vi "Proyecto2.vi"() -> ()   [LabVIEW 2015]
uses:
  <vilib>/Utility/NIReport.llb/image depth.ctl
  <vilib>/MakerHub/LINX/Public/Peripherals/PWM/PWM Set Duty Cycle 1 Chan.vi
  <vilib>/MakerHub/LINX/Public/Peripherals/Digital/Digital Write 1 Chan.vi
  <vilib>/MakerHub/LINX/Public/Peripherals/Digital/Digital Write N Chans.vi
  <vilib>/MakerHub/LINX/Private/Local IO/LinxDigitalWrite.vi
  <vilib>/MakerHub/LINX/Public/Utilities/Check Channel.vi
  <vilib>/MakerHub/LINX/Public/Utilities/Open Serial.vi
  <vilib>/MakerHub/LINX/Public/Peripherals/PWM/PWM Set Duty Cycle N Chans.vi
  <vilib>/MakerHub/LINX/Private/Utilties/Generate Error.vi
  <vilib>/Utility/NIReport.llb/Append Report Text (str wrap).vi
  <vilib>/printing/OpenHTMLReport.llb/Open HTML Report in Browser (Refnum).vi
  <vilib>/Utility/NIReport.llb/NI_report.lvclass
  <vilib>/MakerHub/LINX/LMH-LINX.lvlib
  <vilib>/Utility/NIReport.llb/NI_ReportGenerationCore.lvlib
panel:
  out "Temporary HTML file created":path
  in  "Header":string="Example Report with Images"
  in  "Body":string="<tab>This is an example of some of the things that you can do with HTML reports. <newline> <tab>Above is an image of a Waveform Chart Control.  Below is a horizontal line.  Below that is a link to NI's homepage.<newline>"
  out "Grafica de  distancia entre vehiculo objeto\ndurante el viaje":dbl(graph)
  in  "stop":bool
  out "Velocidad del motor (Escala 0 a 1)":dbl(slide) scale=0.0..1.0
  out "Vehiculo avanzando hacia adelante":bool
  out "Se mantiene a una distancia segura":bool
  out "Precaucion! Bajando a velocidad segura":bool
  out "Distancia entre conductor y vehiculo delantero":dbl
  in  "Echo Pin (DI)":u8
  in  "Trigger":u8
  in  "Serial Port":refnum<visa-resource-name>="N/A"
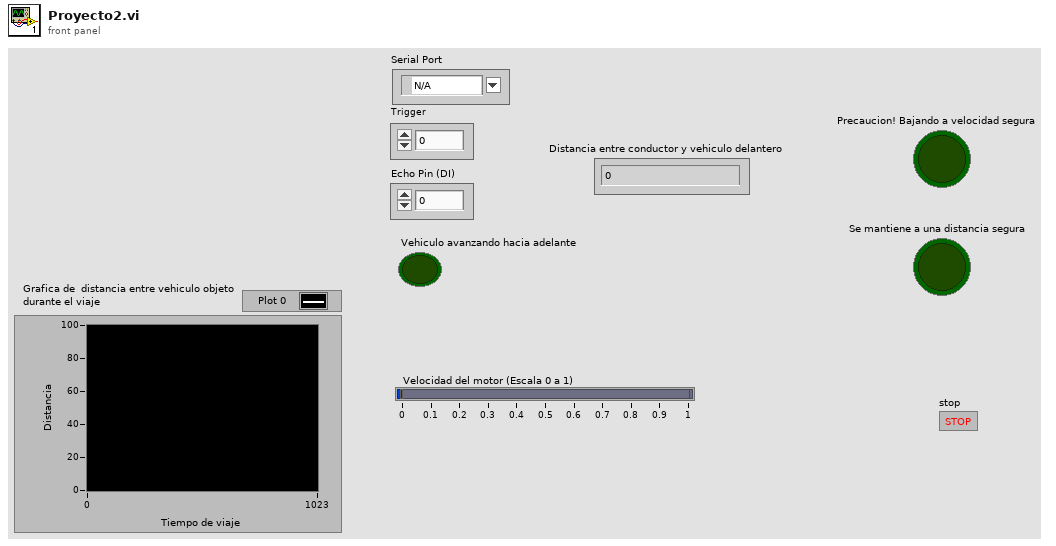
[diagram p1: front panel]
types:
  T1 = typedef "LMH-LINX.lvlib/LINX Ref.ctl" = cluster{"IO":T2, "Interface":T3, "LINX Device Config":T4}
  T2 = typedef "LMH-LINX.lvlib/Platform.ctl" = enum16{"Remote", "Local"}
  T3 = typedef "LMH-LINX.lvlib/Interface.ctl" = enum16{"Serial", "TCP"}
  T4 = typedef "LMH-LINX.lvlib/Device.lvlib/LINX Device Config.ctl" = cluster{"Interface":T3, "COM Port":refnum<visa-resource-name>, "TCP Configuration":T5, "Device Family":u8, "Device ID":u8, "Device Name":string, "TCP Ref":refnum<k5>, "Channels":T6}
  T5 = typedef "LMH-LINX.lvlib/Device.lvlib/TCP Config.ctl" = cluster{"IP Address":string, "Port":u16}
  T6 = typedef "LMH-LINX.lvlib/Channels.ctl" = cluster{"DI":u8[], "DO":u8[], "AI":u8[], "AO":u8[], "PWM":u8[], "QE":u8[], "UART":u8[], "I2C 2":u8[], "SPI":u8[], "CAN":u8[], "Servo":u8[], "AI Ref (V)":dbl, "AI Resolution (Bits)":u8, "AO Ref (V)":dbl, "AO Resolution (Bits)":u8}
  T7 = enum16{"Standard Report", "HTML", "Word", "Excel"}
  T8 = typedef "NI_ReportGenerationCore.lvlib/image depth.ctl" = u16
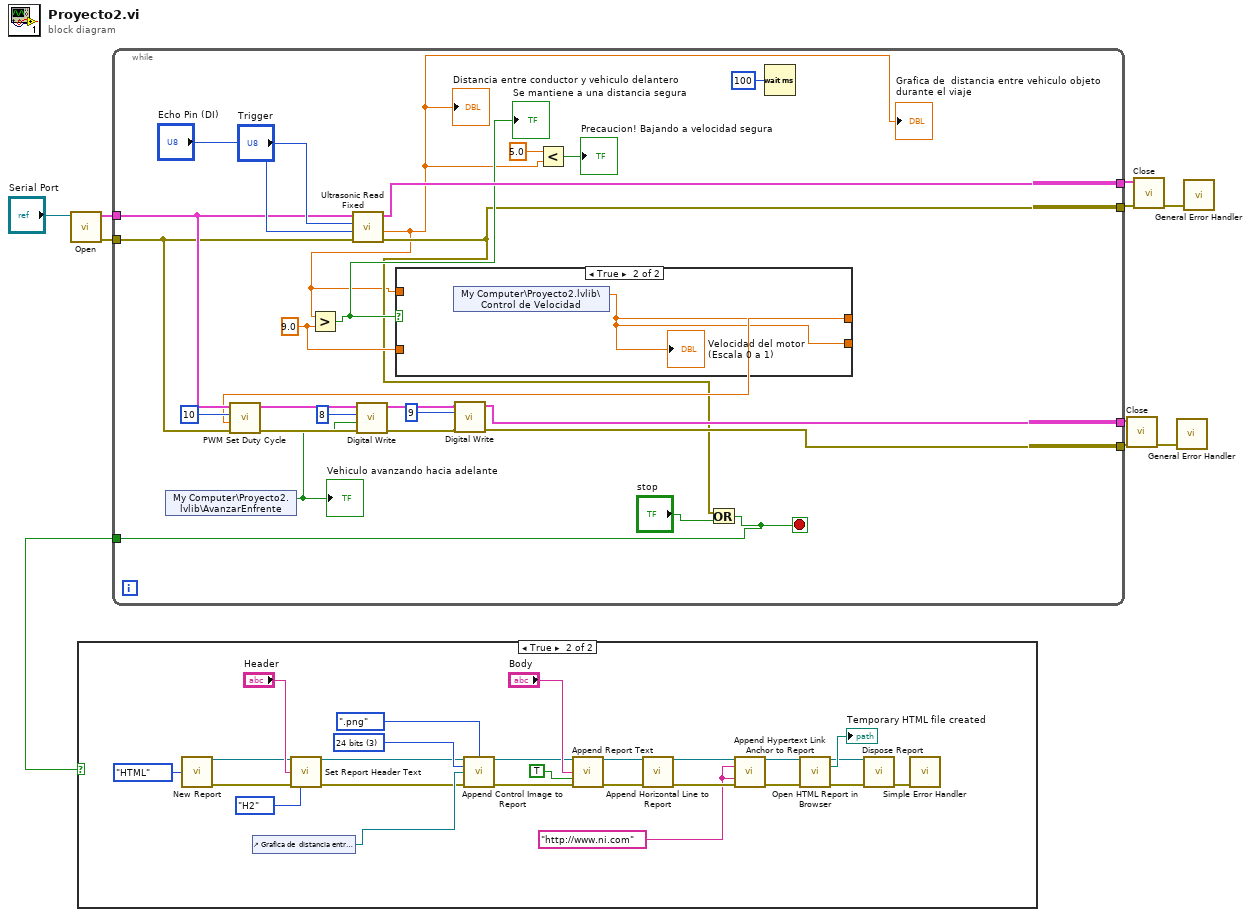
[diagram p0: block diagram]
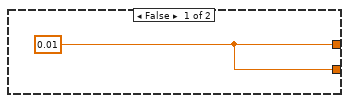
[diagram p3: hidden frame]
diagram:
  n1 = call-poly <vilib>:"Open.vi"("Serial Port"="Serial Port") -> ("Error Out"=w8:errorcluster, "LINX Resource"=w9:T1)  [unwired: 8 in, 1 out]
  n2 = while {
    tunnel: w9 -> [w33]
    tunnel: w8 -> [w32]
    tunnel: [w24] -> w7
    tunnel: [w14] -> w6
    tunnel: [w23] -> w3
    tunnel: [w22] -> w2
    tunnel: [w11] -> w1
    stop <- w11 stop-if-true
    w20 = 9.0 ("y")
    n3 = shared-variable "My Computer\\Proyecto2.lvlib\\AvanzarEnfrente"() -> (w15:bool)  [unwired: 1 in, 1 out]
    "Vehiculo avanzando hacia adelante" <- w15
    n4 = call "Ultrasonic Read Fixed.vi"("Error In"=w32, "DO Channel"="Echo Pin (DI)", "DI Channel"="Trigger", "LINX Resource"=w33) -> ("Error Out"=w14:errorcluster, "Centimeters"=w12:dbl, "LINX Resource"=w24:T1)  [unwired: 4 in, 1 out]
    "Distancia entre conductor y vehiculo delantero" <- w12
    "Grafica de  distancia entre vehiculo objeto\ndurante el viaje" <- w12
    n5 = Greater?(x=w12, y=w20) -> (0:w16:bool)
    "Se mantiene a una distancia segura" <- w16
    n6 = case shown="True" w16 {
      tunnel: w12 -> [_ _]
      tunnel: w20 -> [_ _]
      tunnel: [w36 w37] -> w19
      tunnel: [w36 w37] -> _
      frame False {
        w36 = 0.01
      }
      frame True {
        n7 = shared-variable "My Computer\\Proyecto2.lvlib\\Control de Velocidad"() -> (w37:dbl)  [unwired: 1 in, 1 out]
        "Velocidad del motor (Escala 0 a 1)" <- w37
      }
    }
    n8 = call-poly <vilib>:"PWM Set Duty Cycle.vi"("Error In"=w32, "Duty Cycle (0-1)"=w19, "PWM Channel"=u8 10, "LINX Resource"=w33) -> ("Error Out"=w29:errorcluster, "LINX Resource"=w30:T1)  [unwired: 6 in]
    n9 = call-poly <vilib>:"Digital Write.vi"("Error In"=w29, "Output Value"=w15, "DO Channel"=u8 8, "LINX Resource"=w30) -> ("Error Out"=w28:errorcluster, "LINX Resource"=w27:T1)  [unwired: 6 in]
    n10 = call-poly <vilib>:"Digital Write.vi"("Error In"=w28, "DO Channel"=u8 9, "LINX Resource"=w27) -> ("Error Out"=w22:errorcluster, "LINX Resource"=w23:T1)  [unwired: 7 in]
    n11 = Less?(x=5.0, y=w12) -> (x < y?=→"Precaucion! Bajando a velocidad segura":bool)
    n12 = Or(x=w14, y="stop") -> (x .or. y?=w11:bool)
    n13 = Wait (ms)(milliseconds to wait=u32 100) -> ()  [unwired: 1 out]
  }
  n14 = case shown="True" w1 {
    frame False {
    }
    frame True {
      w58 = T8 3 items=["B&W", "4 bits", "8 bits", "24 bits"] ("image depth")
      w39 = "http://www.ni.com" ("URL of link - href")
      n15 = call <vilib>:"New Report.vi"("report type"=T7."HTML") -> ("report out"=w41:refnum<class "NI_report.lvclass">, "error out"=w40:errorcluster)  [unwired: 13 in]
      n16 = control-ref of="Grafica de  distancia entre vehiculo objeto\ndurante el viaje"() -> (w62:refnum<vi>)
      n17 = call-dynamic "Set Report Header Text.vi"("report in"=w41, "center header text"="Header", "error in (no error)"=w40, "HTML header size"=enum16{"H1", "H2", "H3", "H4", "H5", "H6", "H7"}."H2") -> ("report out"=w50:refnum<class "NI_report.lvclass">, "error out"=w54:errorcluster)  [unwired: 10 in]
      n18 = call-dynamic "Append Control Image to Report.vi"("report in"=w50, "image file type (.jpg)"=enum16{".jpg", ".png"}.".png" ("image file type"), "image depth"=w58, "ctrl reference"=w62, "error in (no error)"=w54) -> ("report out"=w47:refnum<class "NI_report.lvclass">, "error out"=w46:errorcluster)  [unwired: 7 in, 2 out]
      n19 = call-poly <vilib>:"Append Report Text.vi"("report in"=w47, "text"="Body", "append on new line? (F)"=TRUE, "error in (no error)"=w46) -> ("report out"=w48:refnum<class "NI_report.lvclass">, "error out"=w49:errorcluster)  [unwired: 8 in, 2 out]
      n20 = call-dynamic "Append Horizontal Line to Report.vi"("report in"=w48, "error in (no error)"=w49) -> ("report out"=w55:refnum<class "NI_report.lvclass">, "error out"=w56:errorcluster)  [unwired: 12 in]
      n21 = call-dynamic "Append Hypertext Link Anchor to Report.vi"("report in"=w55, "URL of link - href"=w39, "link text"=w39, "error in (no error)"=w56) -> ("report out"=w61:refnum<class "NI_report.lvclass">, "error out"=w60:errorcluster)  [unwired: 8 in, 2 out]
      n22 = call-poly <vilib>:"Open HTML Report in Browser.vi"("report in"=w61, "error in (no error)"=w60) -> ("report out"=w57:refnum<class "NI_report.lvclass">, "temporary HTML file created"=→"Temporary HTML file created":path, "error out"=w38:errorcluster)  [unwired: 11 in]
      n23 = call-dynamic "Dispose Report.vi"("report in"=w57, "error in (no error)"=w38) -> ("error out"=w51:errorcluster)  [unwired: 13 in]
      n24 = call <vilib>:"Simple Error Handler.vi"("error in (no error)"=w51) -> ()  [unwired: 4 in, 5 out]
    }
  }
  n25 = call <vilib>:"Close.vi"("Error In"=w2, "LINX Resource"=w3) -> ("Error Out"=w4:errorcluster)  [unwired: 9 in]
  n26 = call <vilib>:"Close.vi"("Error In"=w6, "LINX Resource"=w7) -> ("Error Out"=w5:errorcluster)  [unwired: 9 in]
  n27 = call <vilib>:"General Error Handler.vi"("error in (no error)"=w4) -> ()  [unwired: 10 in, 5 out]
  n28 = call <vilib>:"General Error Handler.vi"("error in (no error)"=w5) -> ()  [unwired: 10 in, 5 out]
